vi "Generar.vi"() -> ()   [LabVIEW 2021]
uses:
  Global 1.vi
  <vilib>/Analysis/NI_AALBase.lvlib
panel:
  in  "Válvula":bool
  in  "Señal continua":bool
  in  "Ciclo de trabajo":dbl=0.9
  in  "stop 2":bool
  out "Consigna":waveform(dbl)(graph)
  in  "Offset":dbl=0.1 format="%.3f"
  in  "f1":dbl=8.0 format="%0.2p"
  in  "Info. muestreo":cluster{"Fs (Hz)":dbl, "t (s)":dbl}={"Fs (Hz)"=1000.0, "t (s)"=20.0} {"Fs (Hz)" format="%.2p"}
  in  "Fase":dbl format="%.2p"
  in  "Amplitud":dbl=0.05 format="%.3f"
  in  "f0":dbl=0.08 format="%.3f"
  in  "Señal":u16(ring) items=["Senoidal", "Chirp", "Escalón"]
  in  "Comenzar":bool
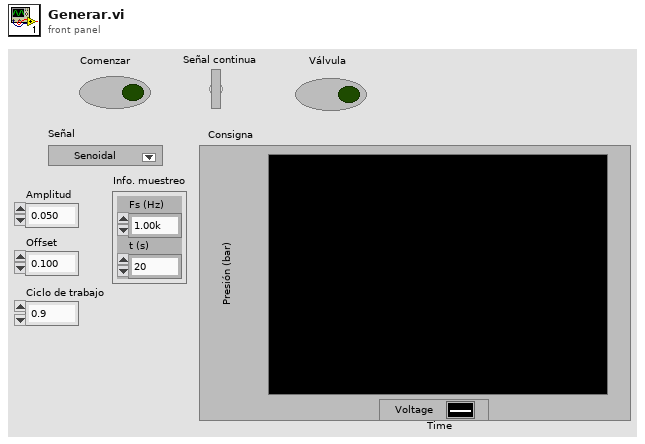
[diagram p1: front panel]
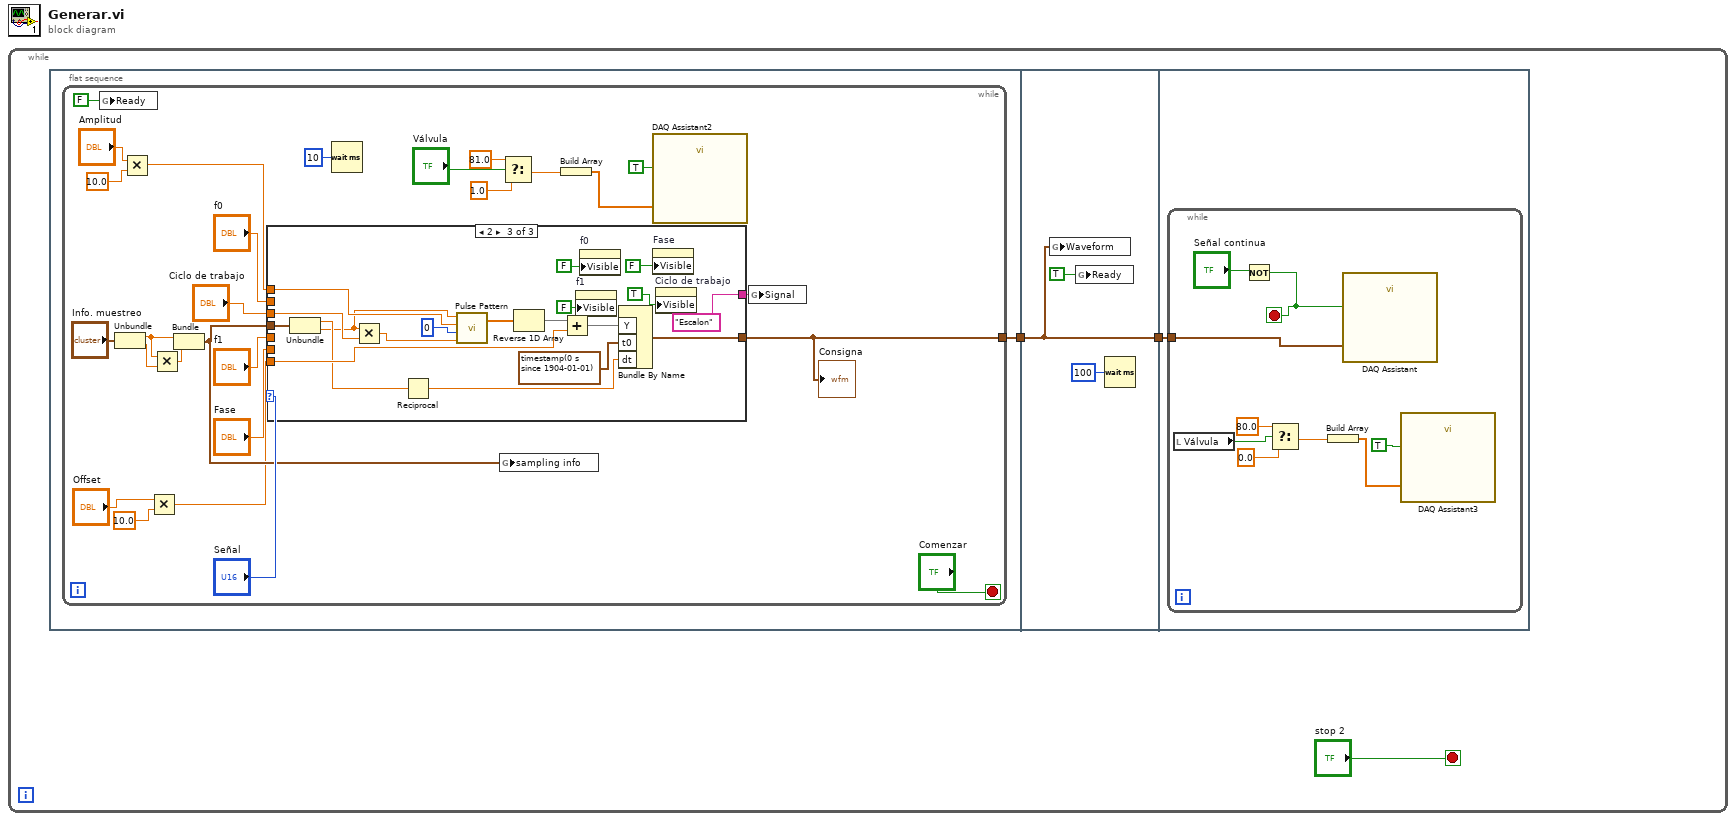
[diagram p0: block diagram]
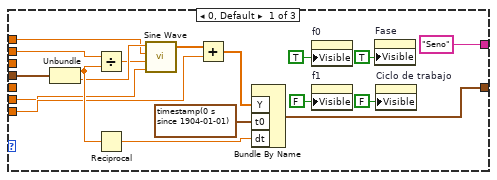
[diagram p2: hidden frame]
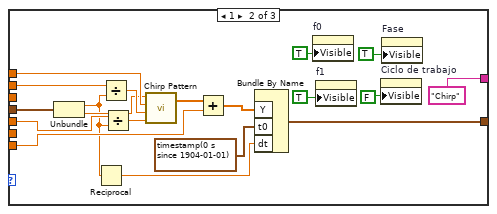
[diagram p3: hidden frame]
diagram:
  n1 = while {
    stop <- "stop 2" stop-if-true
    n2 = flat-sequence {
      tunnel: [w4] -> w2
      tunnel: w2 -> [w90]
      tunnel: [w90] -> w1
      tunnel: w1 -> [w91]
      frame #0 {
        n3 = while {
          tunnel: [w28] -> w4
          stop <- "Comenzar" stop-if-true
          n4 = global write "Global 1.vi" "Ready"(FALSE ("Ready")) -> ()
          n5 = Unbundle("Info. muestreo") -> ("Fs (Hz)"=w8:dbl, "t (s)"=w9:dbl)
          n6 = Multiply(x="Amplitud", y=10.0 ("f")) -> (x*y=w6:dbl)
          n7 = Multiply(x="Offset", y=10.0 ("f")) -> (x*y=w5:dbl)
          n8 = Multiply(x=w8, y=w9) -> (x*y=w11:dbl)
          n9 = Bundle("Fs (Hz)"=w8, w11) -> (w7:cluster{"Fs (Hz)":dbl, dbl})  [unwired: 1 in]
          n10 = case shown="2" "Señal" {
            tunnel: [w45 w58 w86] -> w28
            tunnel: "f0" -> [w43 w64 _]
            tunnel: w6 -> [w40 w68 w82]
            tunnel: "Fase" -> [w38 _ _]
            tunnel: w7 -> [w37 w52 w71]
            tunnel: "f1" -> [_ w65 _]
            tunnel: w5 -> [w44 w66 w77]
            tunnel: "Ciclo de trabajo" -> [_ _ w84]
            tunnel: ["Seno" ("Signal") "Chirp" ("Signal") "Escalon" ("Signal")] -> w24
            frame 0, Default {
              n11 = Unbundle(w37) -> ("Fs (Hz)"=w49:dbl, w41:dbl)
              n12 = Divide(x=w43, y=w49) -> (x/y=w39:dbl)
              n13 = Reciprocal(x=w49) -> (1/x=w47:dbl)
              n14 = call <vilib>:"Sine Wave.vi"("samples"=w41, "amplitude"=w40, "frequency"=w39, "phase in"=w38) -> ("sine wave"=w42:dbl[])  [unwired: 1 in, 2 out]
              n15 = Add(x=w42, y=w44) -> (x+y=w46:dbl[])
              n16 = Bundle By Name("Y"=w46, "t0"=timestamp(0 s since 1904-01-01), "dt"=w47) -> (w45:waveform(dbl))  [unwired: 1 in]
              n17 = property on="f0" class="DigNum (strict)"("Visible"=TRUE) -> ()  [unwired: 2 in, 2 out]
              n18 = property on="f1" class="DigNum (strict)"("Visible"=FALSE) -> ()  [unwired: 2 in, 2 out]
              n19 = property on="Fase" class="DigNum (strict)"("Visible"=TRUE) -> ()  [unwired: 2 in, 2 out]
              n20 = property on="Ciclo de trabajo" class="DigNum (strict)"("Visible"=FALSE) -> ()  [unwired: 2 in, 2 out]
            }
            frame 1 {
              n21 = Unbundle(w52) -> ("Fs (Hz)"=w50:dbl, w51:dbl)
              n22 = Reciprocal(x=w50) -> (1/x=w60:dbl)
              n23 = Divide(x=w64, y=w50) -> (x/y=w63:dbl)
              n24 = Divide(x=w65, y=w50) -> (x/y=w62:dbl)
              n25 = call <vilib>:"Chirp Pattern.vi"("f2"=w62, "f1"=w63, "amplitude"=w68, "samples"=w51) -> ("Chirp Pattern"=w67:dbl[])  [unwired: 1 out]
              n26 = Add(x=w67, y=w66) -> (x+y=w59:dbl[])
              n27 = Bundle By Name("Y"=w59, "t0"=timestamp(0 s since 1904-01-01), "dt"=w60) -> (w58:waveform(dbl))  [unwired: 1 in]
              n28 = property on="f0" class="DigNum (strict)"("Visible"=TRUE) -> ()  [unwired: 2 in, 2 out]
              n29 = property on="f1" class="DigNum (strict)"("Visible"=TRUE) -> ()  [unwired: 2 in, 2 out]
              n30 = property on="Ciclo de trabajo" class="DigNum (strict)"("Visible"=FALSE) -> ()  [unwired: 2 in, 2 out]
              n31 = property on="Fase" class="DigNum (strict)"("Visible"=TRUE) -> ()  [unwired: 2 in, 2 out]
            }
            frame 2 {
              n32 = Unbundle(w71) -> ("Fs (Hz)"=w70:dbl, w69:dbl)
              n33 = Multiply(x=w69, y=w84) -> (x*y=w83:dbl)
              n34 = Reciprocal(x=w70) -> (1/x=w85:dbl)
              n35 = call <vilib>:"Pulse Pattern.vi"("width"=w83, "delay"=0, "amplitude"=w82, "samples"=w69) -> ("Pulse Pattern"=w80:dbl[])  [unwired: 1 out]
              n36 = Reverse 1D Array(array=w80) -> (reversed array=w78:dbl[])
              n37 = Add(x=w78, y=w77) -> (x+y=w76:dbl[])
              n38 = property on="f1" class="DigNum (strict)"("Visible"=FALSE) -> ()  [unwired: 2 in, 2 out]
              n39 = property on="f0" class="DigNum (strict)"("Visible"=FALSE) -> ()  [unwired: 2 in, 2 out]
              n40 = Bundle By Name("Y"=w76, "t0"=timestamp(0 s since 1904-01-01), "dt"=w85) -> (w86:waveform(dbl))  [unwired: 1 in]
              n41 = property on="Fase" class="DigNum (strict)"("Visible"=FALSE) -> ()  [unwired: 2 in, 2 out]
              n42 = property on="Ciclo de trabajo" class="DigNum (strict)"("Visible"=TRUE) -> ()  [unwired: 2 in, 2 out]
            }
          }
          "Consigna" <- w28
          n43 = Wait (ms)(milliseconds to wait=u32 10) -> ()  [unwired: 1 out]
          n44 = global write "Global 1.vi" "sampling info"(w7) -> ()
          n45 = Select(t=81.0, s="Válvula", f=1.0) -> (s? t:f=w18:dbl)
          n46 = Build Array(w18) -> (w17:dbl[])
          n47 = call "DAQ Assistant2"("data"=w17, "stop (T)"=TRUE) -> ()  [unwired: 16 in, 2 out]
          n48 = global write "Global 1.vi" "Signal"(w24) -> ()
        }
      }
      frame #1 {
        n49 = global write "Global 1.vi" "Waveform"(w90) -> ()
        n50 = global write "Global 1.vi" "Ready"(TRUE ("Ready")) -> ()
        n51 = Wait (ms)(milliseconds to wait=u32 100) -> ()  [unwired: 1 out]
      }
      frame #2 {
        n52 = while {
          tunnel: w91 -> [w99]
          stop <- w98 stop-if-true
          n53 = local read "Válvula"() -> (w93:bool)
          n54 = Not(x="Señal continua") -> (.not. x?=w98:bool)
          n55 = Select(t=80.0, s=w93, f=0.0) -> (s? t:f=w95:dbl)
          n56 = Build Array(w95) -> (w94:dbl[])
          n57 = call "DAQ Assistant"("data"=w99, "stop (T)"=w98) -> ()  [unwired: 16 in, 2 out]
          n58 = call "DAQ Assistant3"("data"=w94, "stop (T)"=TRUE) -> ()  [unwired: 16 in, 2 out]
        }
      }
    }
  }
